vi "UTIL_Read_TestVector File.vi"() -> ()   [LabVIEW 2024]
uses:
  Control Definitions/Def FullCfg.ctl
  Control Definitions/Def BenchCfg.ctl
  Control Definitions/Def PumpCtlRefs.ctl
  Control Definitions/Def Bench Status.ctl
  Control Definitions/Ded Spec RNG.ctl
  Control Definitions/Ded LUT_Status.ctl
  Control Definitions/Def Results2.ctl
  <vilib>/Utility/NIReport.llb/Report Type.ctl
  Control Definitions/Def Measure.ctl
  <vilib>/addons/_office/excel.llb/Excel Get Data ([dbl]).vi
  <vilib>/Utility/NIReport.llb/NI_report.lvclass
  <vilib>/Utility/NIReport.llb/Excel/NI_Excel.lvclass
  <vilib>/addons/_office/NI_ReportGenerationToolkit.lvlib
  <vilib>/Utility/NIReport.llb/NI_ReportGenerationCore.lvlib
panel:
  out "Results out":T1=[[{"Fill"=0.0, "Drain"=2.099877125373254, "Status"=8, "Resistor"=100.21026113775098}, {"Fill"=0.0, "Drain"=2.340884884027335, "Status"=8, "Resistor"=100.38318191360392}], [{"Fill"=2.170042696439303, "Drain"=2.5586365748185385, "Status"=8, "Resistor"=230.02559633098178}, {"Fill"=2.382030070818388, "Drain"=2.7907991751157324, "Status"=8, "Resistor"=199.40772021347976}], [{"Fill"=2.602664038291345, "Drain"=2.998016007203322, "Status"=8, "Resistor"=298.43976807060625}, {"Fill"=2.838801735071036, "Drain"=3.2315697490985578, "Status"=8, "Resistor"=256.70779291225386}], [{"Fill"=3.059733787389902, "Drain"=3.4531974906921388, "Status"=8, "Resistor"=397.49638419743775}, {"Fill"=3.2687396024557263, "Drain"=3.677707272016085, "Status"=8, "Resistor"=397.4461284871336}], [{"Fill"=3.509449276263897, "Drain"=3.9038074710552513, "Status"=8, "Resistor"=497.35714487530157}, {"Fill"=3.7240206055274383, "Drain"=4.134181088374212, "Status"=8, "Resistor"=497.0677903515261}], [{"Fill"=3.9513131439502427, "Drain"=4.343285949120155, "Status"=8, "Resistor"=597.5502618369562}, {"Fill"=4.16807129757221, "Drain"=4.577635136824387, "Status"=8, "Resistor"=596.9643842648493}], [{"Fill"=4.62921566273616, "Drain"=4.799759528526893, "Status"=10, "Resistor"=688.3326714430705}, {"Fill"=4.630905126131498, "Drain"=5.013933727264405, "Status"=10, "Resistor"=672.6575275961901}], [{"Fill"=4.868633240626409, "Drain"=5.244008785834679, "Status"=8, "Resistor"=797.8410850665261}, {"Fill"=5.076843846834623, "Drain"=5.469910182659443, "Status"=8, "Resistor"=795.7390467101145}], [{"Fill"=5.681897320087139, "Drain"=5.683090133373554, "Status"=8, "Resistor"=897.3467663579222}, {"Fill"=5.91883022572444, "Drain"=6.0666153846153845, "Status"=8, "Resistor"=896.4714406339958}], [{"Fill"=5.708134947263277, "Drain"=6.439208172724797, "Status"=8, "Resistor"=953.3755132034684}, {"Fill"=6.416548511505127, "Drain"=6.896178876143235, "Status"=8, "Resistor"=996.989267770752}], [{"Fill"=6.175640509385329, "Drain"=0.0, "Status"=8, "Resistor"=1098.2603771455063}, {"Fill"=6.436127330780029, "Drain"=0.0, "Status"=8, "Resistor"=1097.603386419706}]] {"Resistor" format="%.1f"; "Drain" format="%.3f"; "Fill" format="%.3f"}
  in  "aSpec Out":T2[](array[typedef])
  out "Fill!Drain":bool
  in  "Full Config":T4={"Bench Config"={"Name"="OLR001", {"Step Levels"=0.05, "Tolerance"=0.01, "Sample Rate"=0.05, "Resistor"=100.0, "M Level Cal"=1.0, "[B Level Cal"=0.0, "Max Fill Rate"=0.025, "Empty Inches"=8.6, "Full Inches"=2.0}}, "Test Value Table "=[[98.0, 102.0, 7.91, 8.01, 7.55, 7.65, 98.0, 102.0, 7.685, 7.785, 7.325, 7.425], [197.0, 203.0, 7.46, 7.56, 7.1, 7.2, 197.0, 203.0, 7.235, 7.335, 6.875, 6.975], [296.0, 304.0, 7.01, 7.11, 6.65, 6.75, 296.0, 304.0, 6.785, 6.885, 6.425, 6.525], [395.0, 405.0, 6.56, 6.66, 6.2, 6.3, 395.0, 405.0, 6.335, 6.435, 5.975, 6.075], [494.0, 506.0, 6.11, 6.21, 5.75, 5.85, 494.0, 506.0, 5.885, 5.985, 5.525, 5.625], [593.0, 607.0, 5.66, 5.76, 5.3, 5.4, 593.0, 607.0, 5.435, 5.535, 5.075, 5.175], [692.0, 708.0, 5.21, 5.31, 4.85, 4.95, 692.0, 708.0, 4.985, 5.085, 4.625, 4.725], [791.0, 809.0, 4.76, 4.86, 4.4, 4.5, 791.0, 809.0, 4.535, 4.635, 4.175, 4.275], [890.0, 910.0, 4.31, 4.41, 3.95, 4.05, 890.0, 910.0, 4.085, 4.185, 3.725, 3.825], [989.0, 1011.0, 3.86, 3.96, 3.5, 3.6, 989.0, 1011.0, 3.635, 3.735, 3.275, 3.375], [1088.0, 1112.0, 3.41, 3.51, 3.05, 3.15, 1088.0, 1112.0, 3.185, 3.285, 2.825, 2.925], [0.0, 0.0, 0.0, 0.0, 0.0, 0.0, 0.0, 0.0, 0.0, 0.0, 0.0, 0.0]], "Table Col Titles"=[["Aohm Lo", "Aohm Hi", "A Fill Lo", "A Fill Hi", "A Drain Lo", "A Drain Hi", "Bohm Lo", "Bohm Hi", "B Fill Lo", "B Fill Hi", "B Drain Lo", "B Drain Hi"]], "Pump CtlRef In"={"Fill "=refnum, "Drain"=refnum, "Level PV"=refnum, "Flow Rate%"=refnum, "Run Test"=refnum, "Sim"=refnum, "Jog"=refnum, "Level SP"=refnum}, "Bench Status"={"Pump Status"=refnum, "Instrumnet\n Status"=refnum}}
  out "Data":dbl[](array[numeric])=[153.95, 397.7, 397.6, 3.411, 6.210310849633252]
  out "DataQ Input":T8(graph)={"Ch A   Ohms"=397.7, " Ch B  Ohms"=397.6, "Level"=3.411}
  out "Level PV":dbl=6.210310849633252
  out "ChB":dbl=397.6
  out "ChA":dbl=397.7
  out "size(s)":i32[](array[numeric])=[13586, 4]
  in  "Path 2":path=path "C:/Users/ff107/OneDrive/Documents/GitHub/PWC-OLS/$ReportFiles/Vector_Testfile_1.xlsx"
  out "data decimal":dbl[][](array[numeric]) format="%.4f"
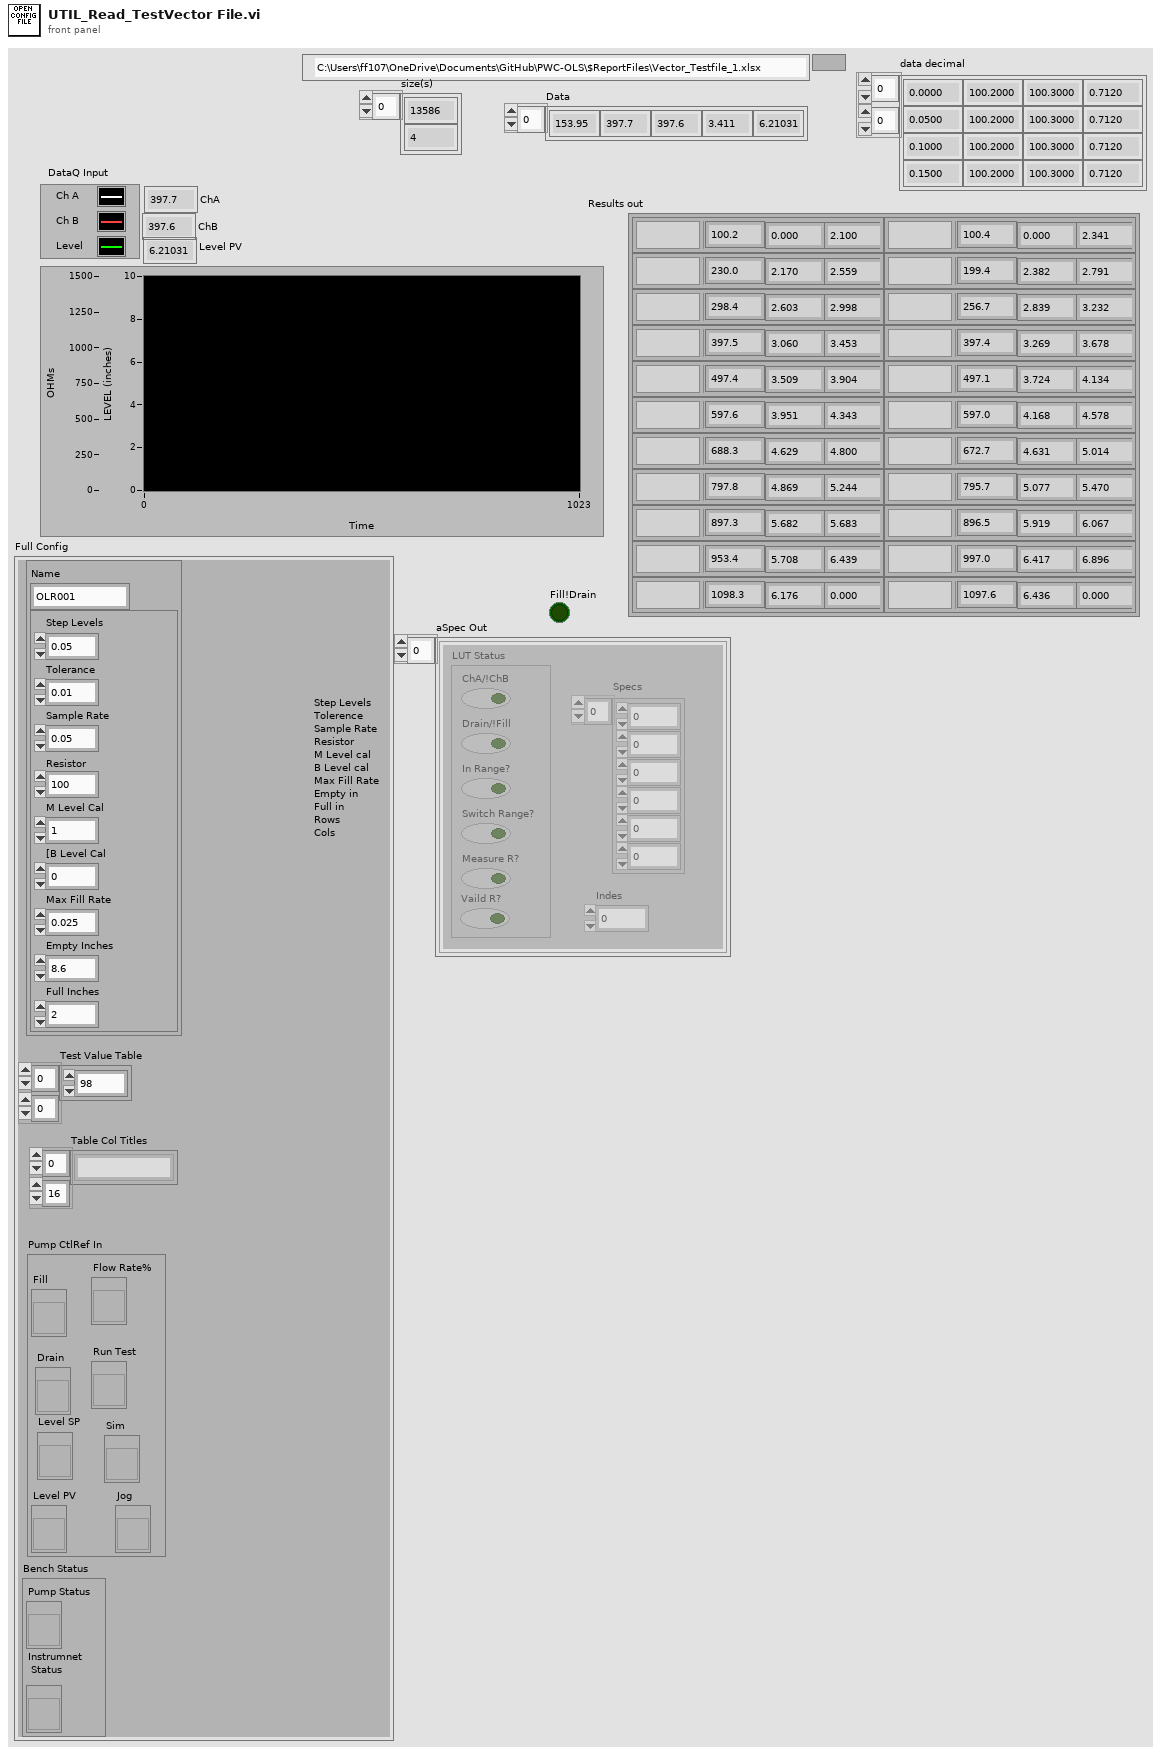
[diagram p1: front panel]
types:
  T1 = typedef "Def Results2.ctl" = cluster{"Fill":dbl, "Drain":dbl, "Status":i16, "Resistor":dbl}[][]
  T2 = typedef "Ded Spec RNG.ctl" = cluster{"Specs":dbl[], "Indes":i32, "LUT Status":T3}
  T3 = typedef "Ded LUT_Status.ctl" = cluster{"ChA/!ChB":bool, "Drain/!Fill":bool, "In Range?":bool, "Switch Range?":bool, "Measure R?":bool, "Vaild R?":bool}
  T4 = typedef "Def FullCfg.ctl" = cluster{"Bench Config":T5, "Test Value Table ":dbl[][], "Table Col Titles":string[][], "Pump CtlRef In":T6, "Bench Status":T7}
  T5 = typedef "Def BenchCfg.ctl" = cluster{"Name":string, cluster{"Step Levels":dbl, "Tolerance":dbl, "Sample Rate":dbl, "Resistor":dbl, "M Level Cal":dbl, "[B Level Cal":dbl, "Max Fill Rate":dbl, "Empty Inches":dbl, "Full Inches":dbl}}
  T6 = typedef "Def PumpCtlRefs.ctl" = cluster{"Fill ":refnum<vi>, "Drain":refnum<vi>, "Level PV":refnum<vi>, "Flow Rate%":refnum<vi>, "Run Test":refnum<vi>, "Sim":refnum<vi>, "Jog":refnum<vi>, "Level SP":refnum<vi>}
  T7 = typedef "Def Bench Status.ctl" = cluster{"Pump Status":refnum<vi>, "Instrumnet\n Status":refnum<vi>}
  T8 = cluster{"Ch A   Ohms":dbl, " Ch B  Ohms":dbl, "Level":dbl}
  T9 = cluster{"Resistor":dbl, "Fill":dbl, "Drain":dbl, "Status":i16}
  T10 = typedef "Def Measure.ctl" = cluster{"ChA R":dbl, "ChB R":dbl, "Level PV":dbl}
  T11 = typedef "NI_ReportGenerationCore.lvlib/Report Type.ctl" = enum16{"HTML", "Word", "Excel"}
  T12 = cluster{"Resistor":dbl, "Fill":dbl, "Drain":dbl, "Status":i16}[][]
  T13 = typedef "Def Xresult.ctl" = cluster{"Switched":bool, "In Range":bool, "Index":i16, "Level OUt":dbl, " Ch n Ohms":dbl, "Drain!Fill":bool}[]
  T14 = cluster{"Ch A   Ohms":dbl, " Ch B  Ohms":dbl, "Level OUt":dbl}
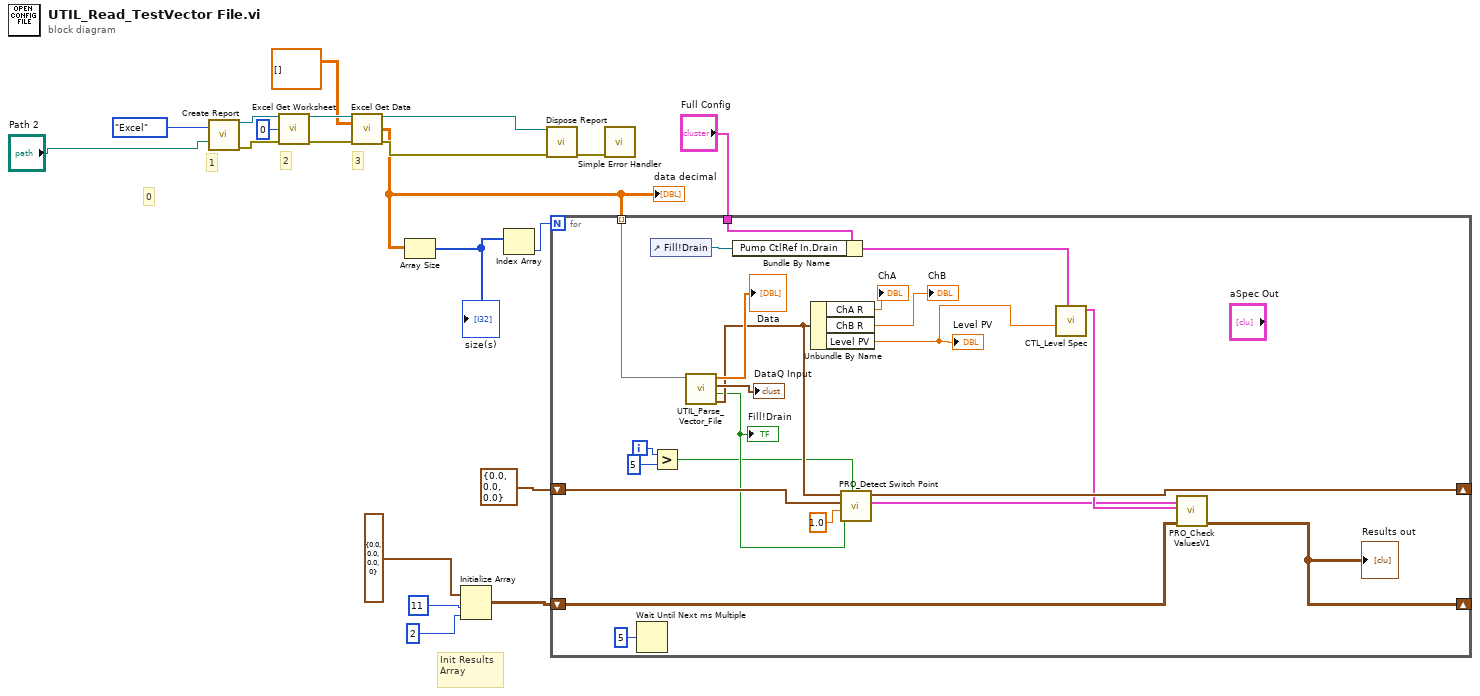
[diagram p0: block diagram]
diagram:
  # "Init Results\nArray"
  # "0"
  # "3"
  # "2"
  # "1"
  n1 = call <vilib>:"Create Report.vi"("report type"=Report_Type."Excel", "template (empty)"="Path 2") -> ("report out"=w16:refnum<class "NI_report.lvclass">, "error out"=w15:errorcluster)  [unwired: 12 in]
  n2 = call <vilib>:"Excel Get Worksheet.vi"("report in"=w16, "worksheet index (0)"=0, "error in (no error)"=w15) -> ("report out"=w18:refnum<class "NI_report.lvclass">, "error out"=w19:errorcluster)  [unwired: 11 in]
  n3 = call-poly <vilib>:"Excel Get Data.vi"("report in"=w18, "data type"=dbl[][] [], "error in (no error)"=w19) -> ("report out"=w11:refnum<class "NI_report.lvclass">, "data"=w7:dbl[][], "error out"=w10:errorcluster)  [unwired: 10 in]
  "data decimal" <- w7
  n4 = Array Size(array=w7) -> (size(s)=w9:i32[])
  "size(s)" <- w9
  n5 = Initialize Array(T9 {"Resistor"=0.0, "Fill"=0.0, "Drain"=0.0, "Status"=0} ("Cluster 2"), 11 ("dimension size"), 2 ("dimension size")) -> (w1:T12)
  n6 = Index Array(array=w9) -> (element=w8:i32)  [unwired: 1 in]
  n7 = call-dynamic "Dispose Report.vi"("report in"=w11, "error in (no error)"=w10) -> ("error out"=w12:errorcluster)  [unwired: 13 in]
  n8 = for {
    N: w8 -> [_]
    tunnel: w7 -> [w40] mode=indexing
    tunnel: "Full Config" -> [w39]
    shift-right: [w31] -> _
    shift-left: T10 {"ChA R"=0.0, "ChB R"=0.0, "Level PV"=0.0} ("Measure") -> [w33]
    shift-right: [w27] -> _
    shift-left: w1 -> [w26]
    i -> [w24]
    n9 = Wait Until Next ms Multiple(millisecond multiple=u32 5) -> ()  [unwired: 1 out]
    n10 = control-ref of="Fill!Drain"() -> (w38:refnum<vi>)
    n11 = Greater?(x=w24, y=5) -> (0:w22:bool)
    n12 = call "UTIL_Parse_Vector_File.vi"("data"=w40) -> ("Measure"=w32:T10, "Drain!Fill"=w25:bool, "Cluster"=→"DataQ Input":cluster{dbl, dbl, dbl}, "Array"=→"Data":dbl[])  [unwired: 7 in]
    "Fill!Drain" <- w25
    n13 = Bundle By Name(cluster=w39, "Pump CtlRef In.Drain"=w38) -> (w30:T4)
    n14 = Unbundle By Name(w32) -> ("ChA R"=→"ChA":dbl, "ChB R"=→"ChB":dbl, "Level PV"=w28:dbl)
    "Level PV" <- w28
    n15 = call "PRO_Detect Switch Point.vi"("Enable"=w22, "Drain!Fill"=w25, "Fitler TC"=1.0, "Measure N-1"=w33, "Measure N"=w32) -> ("XResult"=w21:T13, "Measure N out"=w31:T14)  [unwired: 2 in, 3 out]
    n16 = call "CTL_Level Spec.vi"("Full Config"=w30, "Level IN inches"=w28) -> ("aSpec Out"=w29:T2[])  [unwired: 8 in, 1 out]
    n17 = call "PRO_Check ValuesV1.vi"("Results in"=w26, "aSpec In"=w29, "Measurement"=w21) -> ("Results out"=w27:T1)  [unwired: 7 in, 1 out]
    "Results out" <- w27
  }
  n18 = call <vilib>:"Simple Error Handler.vi"("error in (no error)"=w12) -> ()  [unwired: 4 in, 5 out]
